vi "Obis Send Command.vi"(0 "VISA Ref":refnum<visa-resource-name>, 7 "Error In":errorcluster, 11 "Command":string) -> (4 "VISA Ref Out":refnum<visa-resource-name>, 8 "Error Out":errorcluster, 15 "Response":string)   [LabVIEW 2020]
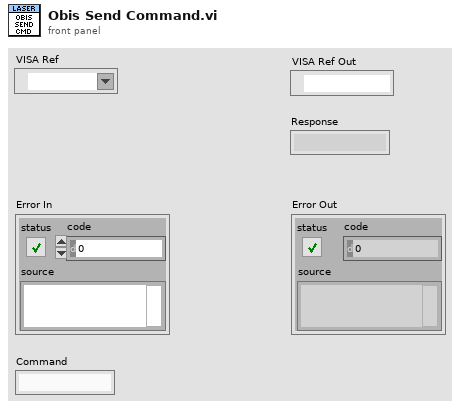
[diagram p1: front panel]
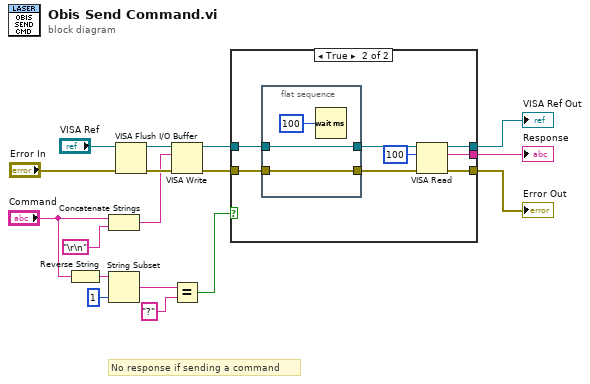
[diagram p0: block diagram]
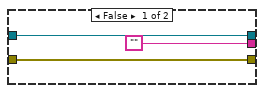
[diagram p2: hidden frame]
diagram:
  # "No response if sending a command"
  n1 = Reverse String(1:"Command") -> (0:w6:string)
  n2 = Concatenate Strings("Command", "\r\n") -> (w7:string)
  n3 = String Subset(string=w6, length (rest)=1 ("length (rest)")) -> (substring=w4:string)  [unwired: 1 in]
  n4 = VISA Flush I/O Buffer(VISA resource name="VISA Ref", error in (no error)="Error In") -> (VISA resource name out=w10:refnum<visa-resource-name>, error out=w11:errorcluster)  [unwired: 1 in]
  n5 = VISA Write(VISA resource name=w10, write buffer=w7, error in (no error)=w11) -> (VISA resource name out=w17:refnum<visa-resource-name>, error out=w16:errorcluster)  [unwired: 1 out]
  n6 = Equal?(x=w4, y="?") -> (x = y?=w1:bool)
  n7 = case shown="True" w1 {
    tunnel: w17 -> [w18 w28]
    tunnel: w16 -> [w20 w24]
    tunnel: [w18 w27] -> w15
    tunnel: [w20 w26] -> w14
    tunnel: ["" w25] -> w13
    frame False {
    }
    frame True {
      n8 = flat-sequence {
        tunnel: [w30] -> w22
        tunnel: w28 -> [w30]
        tunnel: [w29] -> w23
        tunnel: w24 -> [w29]
        frame #0 {
          n9 = Wait (ms)(milliseconds to wait=u32 100) -> ()  [unwired: 1 out]
        }
      }
      n10 = VISA Read(VISA resource name=w22, byte count=u32 100, error in (no error)=w23) -> (VISA resource name out=w27:refnum<visa-resource-name>, read buffer=w25:string, error out=w26:errorcluster)  [unwired: 1 out]
    }
  }
  "Response" <- w13
  "VISA Ref Out" <- w15
  "Error Out" <- w14
